vi "Pulse - Set Transient and Width.vi"(8 "error in (no error)":errorcluster, 10 "Trigger Settings":T1, 11 "3300 in":refnum<class "3300.lvclass">) -> (0 "error out":errorcluster, 3 "3300 out":refnum<class "3300.lvclass">)   [LabVIEW 2019, in "3300.lvlib" / "3300.lvclass"]
uses:
  Library/3300.lvclass
  C:/Users/Public/Documents/Development/builds/Instruments/Electronic Load.lvlibp/Library/Electronic Load.lvclass
  builds/Instruments/Electronic Load.lvlibp/Custom Controls/Trigger Settings.ctl
  builds/Instruments/Electronic Load.lvlibp/Custom Controls/E-Load Mode.ctl
  Library/3300.lvclass/3300.ctl
  Accessors/Read Local Resource.vi
  Accessors/Write Local Resource.vi
  builds/Instruments/Electronic Load.lvlibp/Accessors/Trigger/Read Pulse Enable.vi
  builds/Instruments/Electronic Load.lvlibp/Accessors/Read Active Channel.vi
  <instrlib>/Agilent N330X Series/Agilent N330X Series.lvlib
  builds/Instruments/Electronic Load.lvlibp/Library/Electronic Load.lvclass
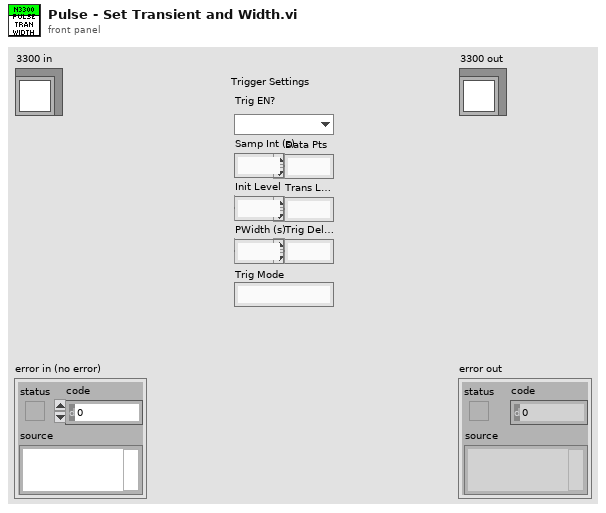
[diagram p1: front panel]
types:
  T1 = typedef "Electronic Load.lvlibp/Electronic Load.lvclass/Trigger Settings.ctl" = cluster{"Mode":T2, "Initial":dbl, "Transient":dbl, "Interval":dbl, "Width":dbl, "Delay":dbl, "Data Pts":i32, "Slew Rate":dbl}
  T2 = typedef "Electronic Load.lvlibp/Electronic Load.lvclass/E-Load Mode.ctl" = enum16{"Current", "Resistance", "Voltage"}
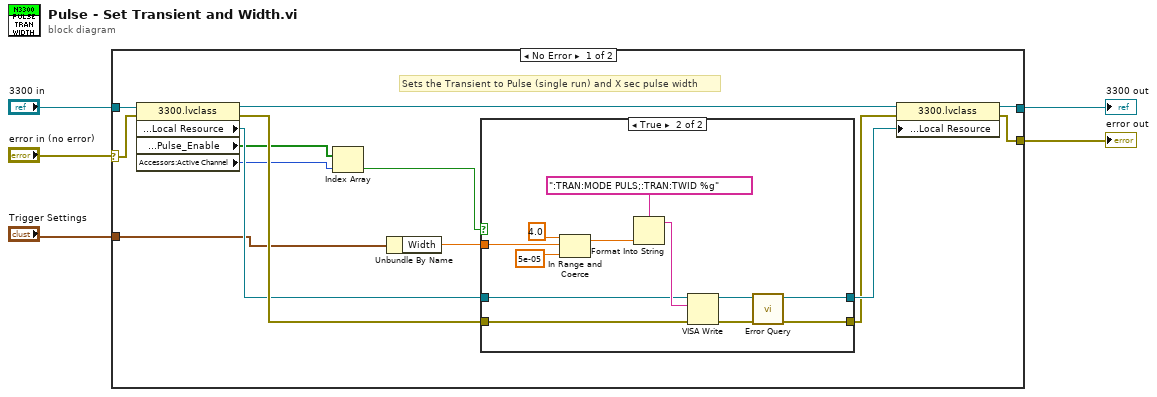
[diagram p0: block diagram]
diagram:
  n1 = case shown="No Error" "error in (no error)" {
    selector: "error in (no error)" -> [w19 w35]
    tunnel: [w13 w35] -> w3
    tunnel: [w17 w34] -> w4
    tunnel: "3300 in" -> [w11 w34]
    tunnel: "Trigger Settings" -> [w9 _]
    frame No Error {
      # "Sets the Transient to Pulse (single run) and X sec pulse width"
      n2 = property class="3300.lvclass"(reference=w11, error in=w19) -> (reference out=w16:refnum<class "3300.lvclass">, error out=w18:errorcluster, "Private:Accessors:Local Resource"=w12:refnum<visa-resource-name>, "Accessors:Settings:Pulse:Pulse_Enable"=w8:bool[], "Accessors:Active Channel"=w7:u32)
      n3 = Index Array(array=w8, index=w7) -> (element=w6:bool)
      n4 = Unbundle By Name(w9) -> ("Width"=w10:dbl)
      n5 = case shown="True" w6 {
        tunnel: w18 -> [w20 w30]
        tunnel: [w21 w29] -> w15
        tunnel: [w20 w28] -> w14
        tunnel: w12 -> [w21 w27]
        tunnel: w10 -> [_ w23]
        frame False {
        }
        frame True {
          n6 = In Range and Coerce(upper limit=4.0, x=w23, lower limit=5e-05) -> (coerced(x)=w22:dbl)  [unwired: 1 out]
          n7 = Format Into String(format string=":TRAN:MODE PULS;:TRAN:TWID %g" ("string (\"\")"), w22) -> (resulting string=w31:string)  [unwired: 2 in, 1 out]
          n8 = VISA Write(VISA resource name=w27, write buffer=w31, error in (no error)=w30) -> (VISA resource name out=w33:refnum<visa-resource-name>, error out=w32:errorcluster)  [unwired: 1 out]
          n9 = call <instrlib>:"Error Query.vi"("error in (no error)"=w32, "VISA resource name"=w33) -> ("error out"=w28:errorcluster, "VISA resource name out"=w29:refnum<visa-resource-name>)  [unwired: 6 in, 2 out]
        }
      }
      n10 = property class="3300.lvclass"(reference=w16, error in=w14, "Private:Accessors:Local Resource"=w15) -> (reference out=w17:refnum<class "3300.lvclass">, error out=w13:errorcluster)
    }
    frame Error {
    }
  }
  "error out" <- w3
  "3300 out" <- w4
